vi "trim_hex_prefix.vi"(1 "string in":string) -> (0 "string out":string)   [LabVIEW 2010]
doc: "This function removes any whitespace and the \"0x\" or \"0X\" hex prefix from a string."
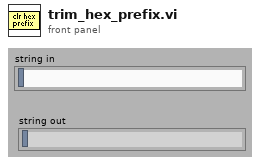
[diagram p1: front panel]
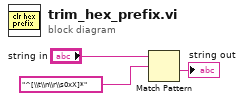
[diagram p0: block diagram]
diagram:
  n1 = Match Pattern(string="string in", regular expression="^[\\t\\n\\r\\s0xX]*") -> (after substring=→"string out":string)  [unwired: 1 in, 3 out]
